vi "gxml_ConcatGXMLStrings.vi"(8 "error in":errorcluster, 10 "GXML Strings":string[](array[string])) -> (0 "error out":errorcluster, 2 "Concatenated GXML String":string)   [LabVIEW 2011, in "Third Party VIs.lvlib" / "GXML.lvlib"]
doc: "This VI concatenates multiple GXML strings into one XML string.\n\nXML specifications say there can only be one top level element in an XML string. This VI concatenates multiple GXML strings inside one <GXML_Root> element."
uses:
  GXML.lvlib
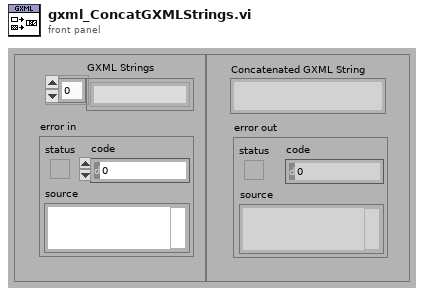
[diagram p1: front panel]
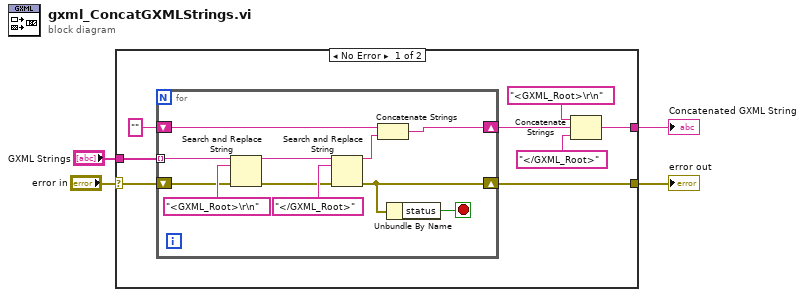
[diagram p0: block diagram]
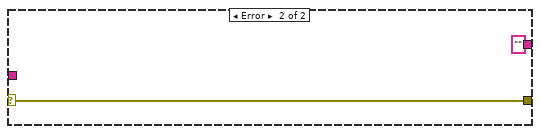
[diagram p2: hidden frame]
diagram:
  n1 = case shown="No Error" "error in" {
    selector: "error in" -> [w6 w25]
    tunnel: "GXML Strings" -> [w12 _]
    tunnel: [w7 ""] -> w3
    tunnel: [w5 w25] -> w1
    frame No Error {
      n2 = for {
        tunnel: w12 -> [w23] mode=indexing
        shift-right: [w17] -> w10
        shift-left: "" -> [w19]
        shift-right: [w14] -> w5
        shift-left: w6 -> [w16]
        stop <- w13 stop-if-true
        n3 = Search and Replace String(input string=w23, search string="<GXML_Root>\r\n", error in=w16) -> (result string=w21:string, error out=w15:errorcluster)  [unwired: 5 in, 2 out]
        n4 = Search and Replace String(input string=w21, search string="</GXML_Root>", error in=w15) -> (result string=w18:string, error out=w14:errorcluster)  [unwired: 5 in, 2 out]
        n5 = Concatenate Strings(w19, w18) -> (w17:string)
        n6 = Unbundle By Name(w14) -> ("status"=w13:bool)
      }
      n7 = Concatenate Strings("<GXML_Root>\r\n", w10, "</GXML_Root>") -> (w7:string)
    }
    frame Error {
    }
  }
  "Concatenated GXML String" <- w3
  "error out" <- w1
